vi "Проект квадроКОПТЕР для сравнения.vi"() -> ()   [LabVIEW 2013]
uses:
  <vilib>/Instr/_visa.llb/VISA Configure Serial Port (Instr).vi
  MadgwickOrientationFilter.lvlib
  <vilib>/picture/3D Picture Control/NI_3D Picture Control.lvlib
panel:
  out "Error":u8
  in  "VISA resource name":refnum<visa-resource-name>="COM5"
  out "cluster 2":T1
  out "Error 5":u8 caption="Error"
  in  "Tab Control":enum32{"3D", "Graphs", "U & I", "Out"}(tab)
  out "Scene Display 2":refnum<vi>(3d-picture)
  out "Scene Display":refnum<vi>(3d-picture)
  out "Кватернион":T1(graph)
  out "Q0":sgl
  out "Q1":sgl
  out "Q2":sgl
  out "Q3":sgl
  out "Boolean":bool
  in  "f_cut_diff_vel_xy":dbl
  in  "f_cut_diff_vel_xy b":bool
  in  "f_cut_err_vel_xy":dbl
  in  "f_cut_err_vel_xy b":bool
  in  "KP_Pos_xy b":bool
  in  "KP_Pos_xy":dbl
  in  "KP_Vel_xy b":bool
  in  "KP_Vel_xy":dbl
  in  "KD_Vel_xy":bool
  in  "KD_Vel_xy":dbl
  in  "KI_Acc_xy b":bool
  in  "KI_Vel_xy":dbl
  in  "f_cut_diff_vel_alt":dbl
  in  "f_cut_diff_vel_alt b":bool
  in  "f_cut_err_vel_alt":dbl
  in  "f_cut_diff_acc_alt b":bool
  in  "KI_ugol_z":dbl
  in  "KI_ugol_z_b":bool
  in  "KP_ugol_z":dbl
  in  "KP_ugol_z_b":bool
  in  "KI_rate_z":dbl
  in  "KI_vel_z_b":bool
  in  "KP_rate_z":dbl
  in  "KP_vel_z_b":bool
  in  "KD_rate_z":dbl
  in  "KD_vel_z_b":bool
  in  "KD_vel_xy_b":bool
  in  "KD_rate_xy":dbl
  in  "KI_vel_xy_b":bool
  in  "KP_vel_xy_b":bool
  in  "KI_rate_xy":dbl
  in  "KP_rate_xy":dbl
  in  "KI_ugla_xy_b":bool
  in  "KP_ugla_xy_b":bool
  in  "KI_ugla_xy":dbl
  in  "KP_ugla_xy":dbl
  in  "f_cut_diff":dbl
  in  "f_cut_diff_b":bool
  in  "KP_Pos_alt b":bool
  in  "KP_Pos_alt":dbl
  in  "KP_Vel_alt b":bool
  in  "KP_Vel_alt":dbl
  in  "KD_Vel_alt b":bool
  in  "KD_Vel_alt":dbl
  in  "KP_Acc_alt b":bool
  in  "KP_Acc_alt":dbl
  in  "KI_Acc_alt b":bool
  in  "KI_Vel_alt":dbl
  in  "KD_Acc_alt b":bool
  in  "KD_Acc_alt":dbl
  out "*(type *) &x 11":sgl
  out "*(type *) &x 10":sgl
  out "*(type *) &x 9":sgl
  out "*(type *) &x 8":sgl
  out "sqrt(x)":dbl
  out "unsigned byte array":u8[](array[numeric])
  out "String":string
  out "*(type *) &x 13":sgl
  out "*(type *) &x 12":sgl
  out "*(type *) &x 7":sgl
  out "*(type *) &x 6":sgl
  out "decimated array":u8[](array[numeric])
  out "*(type *) &x 5":sgl
  out "cluster":T1
  in  "stop":bool
  # "346346"
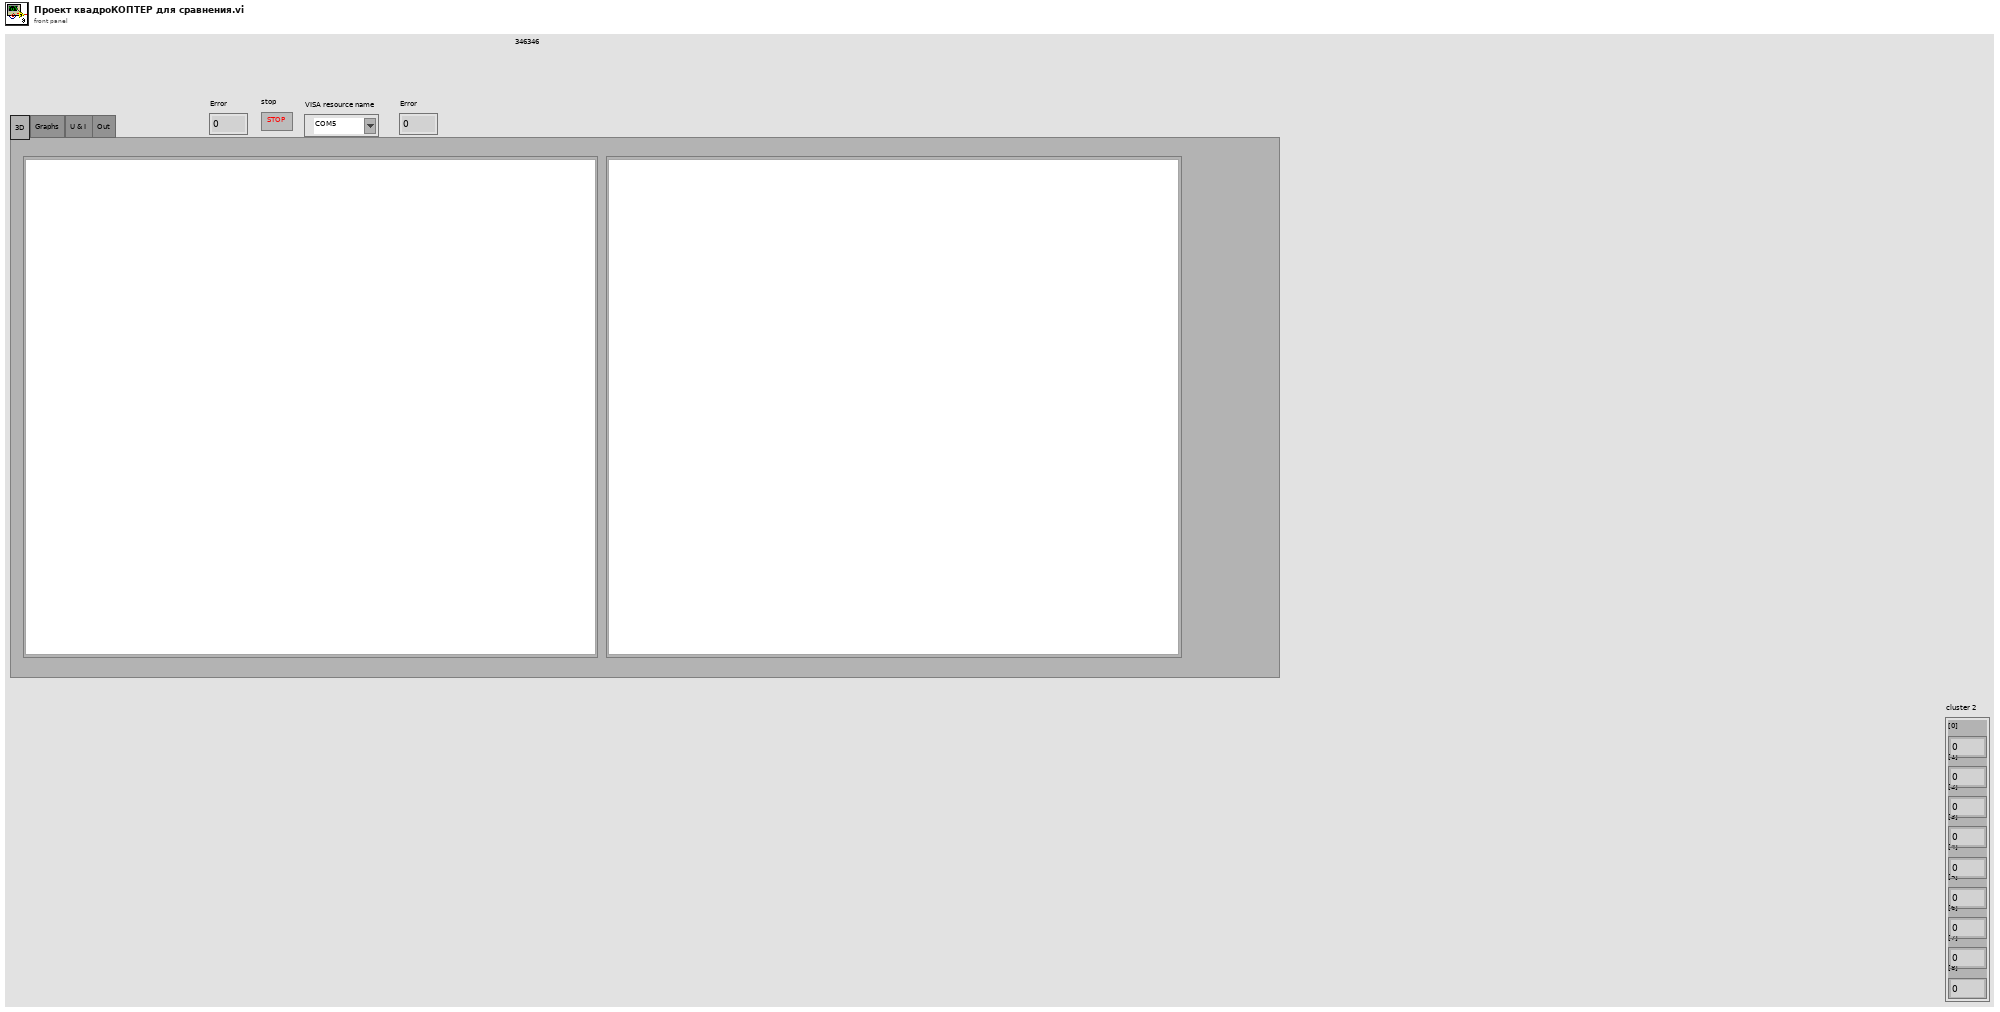
[diagram p1: front panel]
types:
  T1 = cluster{"[0]":dbl, "[1]":dbl, "[2]":dbl, "[3]":dbl, "[4]":dbl, "[5]":dbl, "[6]":dbl, "[7]":dbl, "[8]":dbl}
  T2 = enum16{"open", "replace", "create", "open or create", "replace or create", "replace or create with confirmation"}
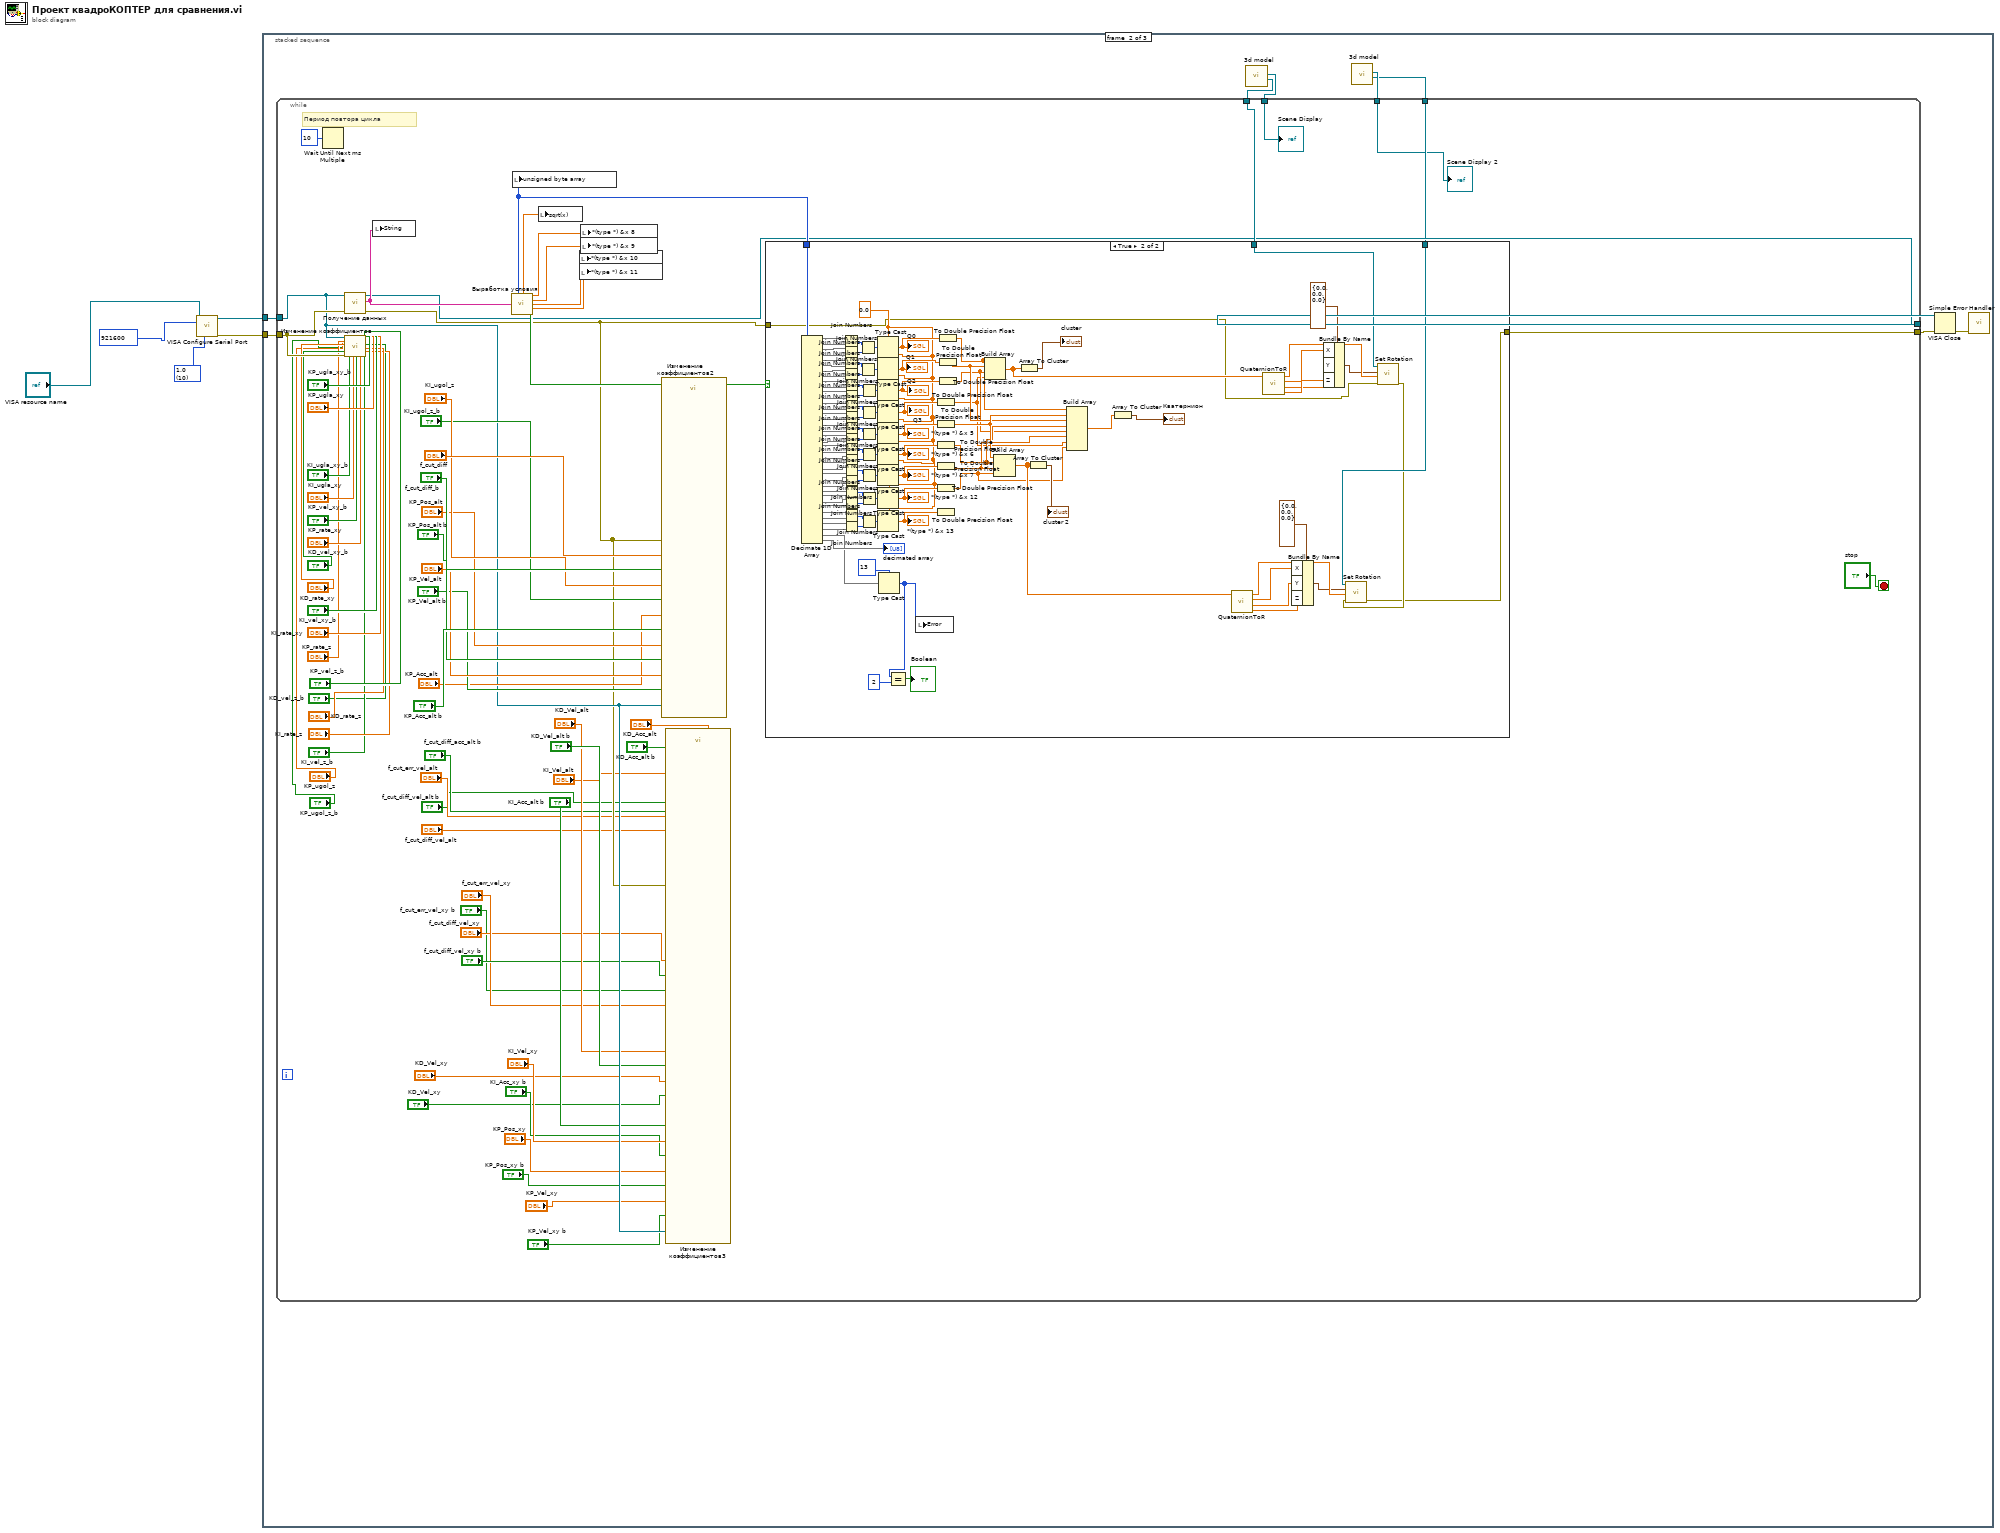
[diagram p0: block diagram]
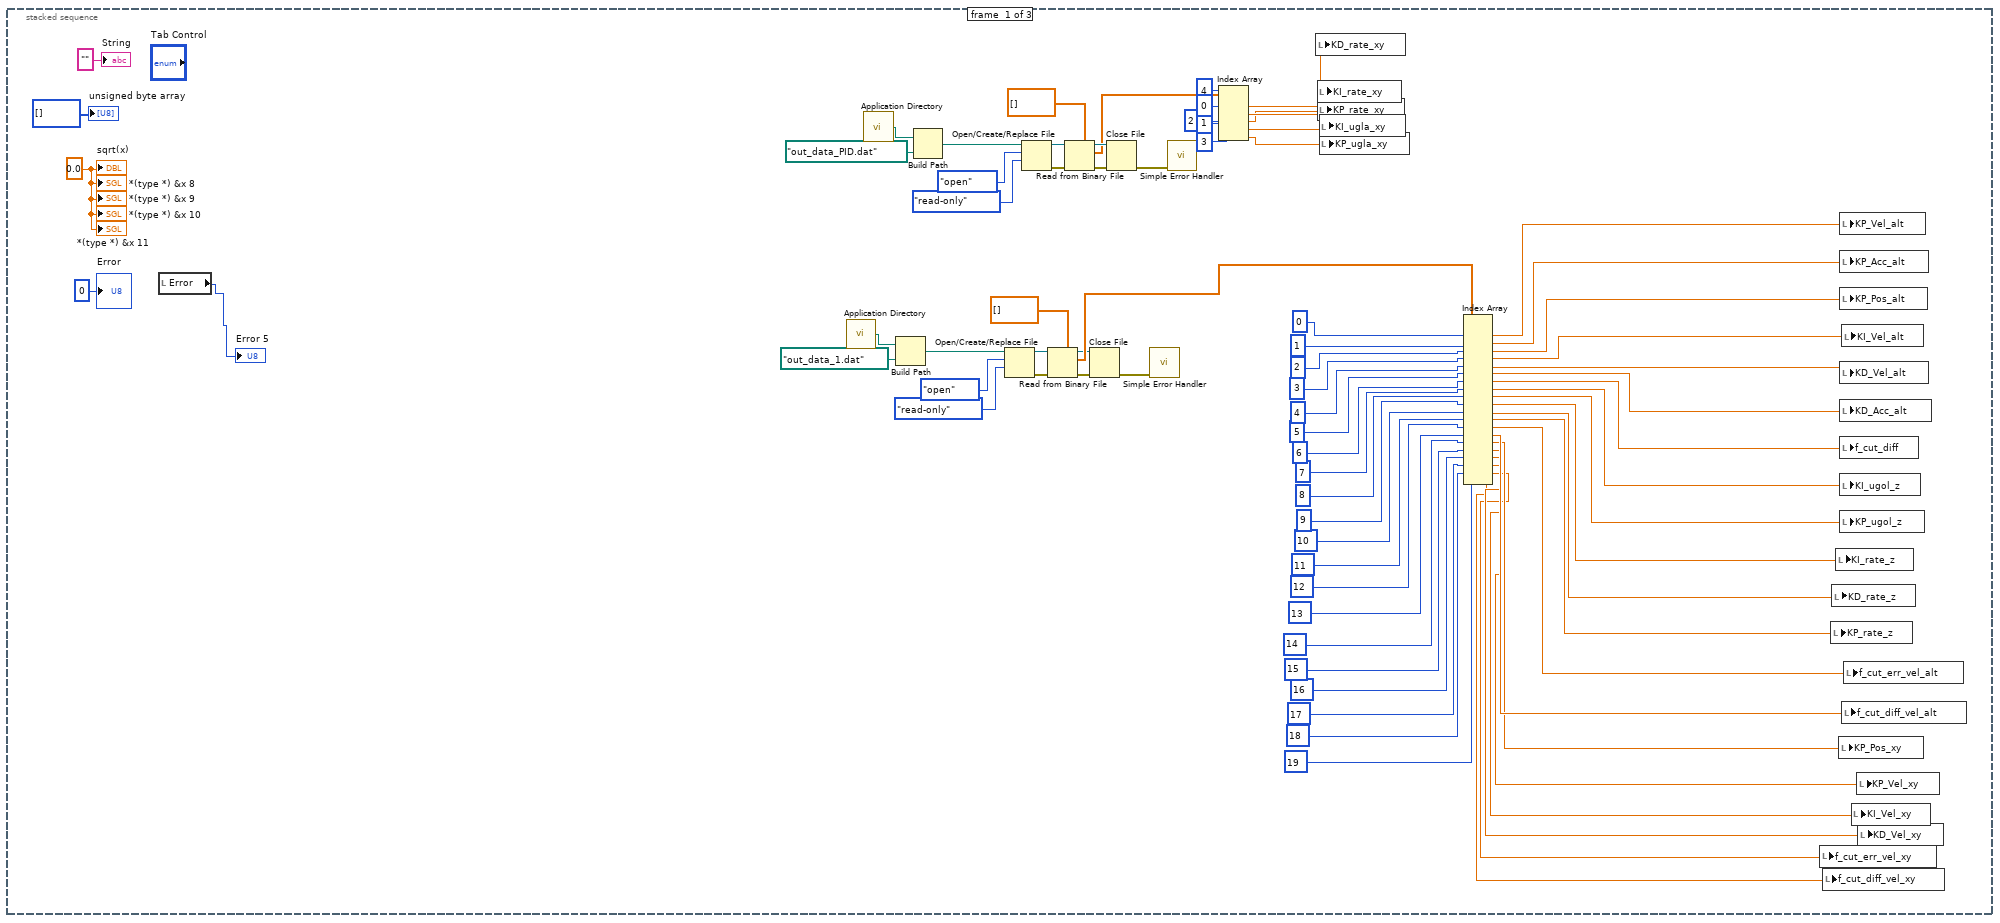
[diagram p2: hidden frame]
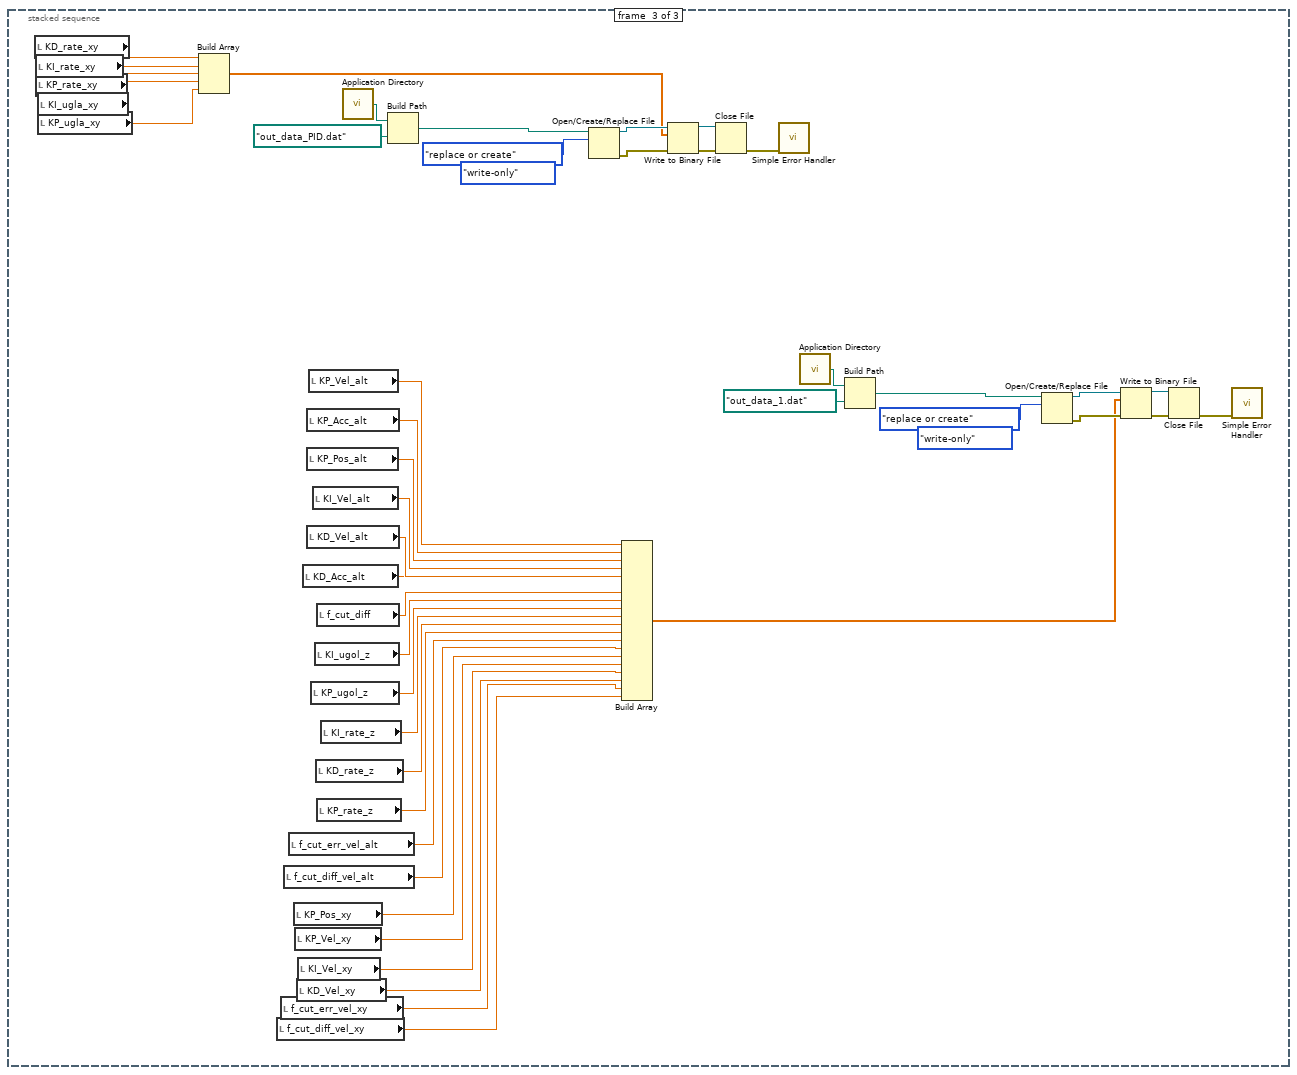
[diagram p4: hidden frame]
diagram:
  w3 = u16 10 items=["1.0"=10, "1.5"=15, "2.0"=20] ("stop bits (10: 1 bit)")
  n1 = call-poly "VISA Configure Serial Port"("VISA resource name"="VISA resource name", "baud rate (9600)"=u32 921600, "stop bits (10: 1 bit)"=w3) -> ("VISA resource name out"=w5:refnum<visa-resource-name>, "error out"=w4:errorcluster)  [unwired: 11 in]
  n2 = stacked-sequence {
    tunnel: w5 -> [_ w93 _]
    tunnel: w4 -> [_ w91 _]
    frame #0 {
      w82 = 0.0 ("sqrt(x)")
      n3 = local read "Error"() -> (→"Error 5":u8)
      n4 = call <vilib>:"Application Directory.vi"() -> ("Application Directory"=w56:path)
      n5 = call <vilib>:"Application Directory.vi"() -> ("Application Directory"=w74:path)
      n6 = Build Path(base path=w56, name or relative path=path "out_data_1.dat" ("default name")) -> (appended path=w52:path)
      n7 = Build Path(base path=w74, name or relative path=path "out_data_PID.dat" ("default name")) -> (appended path=w78:path)
      n8 = Open/Create/Replace File(file path (use dialog)=w52, operation (0:open)=T2."open", access (0:read/write)=enum16{"read/write", "read-only", "write-only"}."read-only") -> (refnum out=w57:refnum<file>, error out=w58:errorcluster)  [unwired: 3 in, 1 out]
      n9 = Open/Create/Replace File(file path (use dialog)=w78, operation (0:open)=T2."open", access (0:read/write)=enum16{"read/write", "read-only", "write-only"}."read-only") -> (refnum out=w73:refnum<file>, error out=w72:errorcluster)  [unwired: 3 in, 1 out]
      n10 = Read from Binary File(5:dbl[] [] ("appended array"), 8:w58, 11:w57) -> (0:w60:errorcluster, 2:w62:dbl[], 3:w59:refnum<file>)  [unwired: 3 in, 1 out]
      n11 = Read from Binary File(5:dbl[] [] ("appended array"), 8:w72, 11:w73) -> (0:w70:errorcluster, 2:w68:dbl[], 3:w71:refnum<file>)  [unwired: 3 in, 1 out]
      n12 = Close File(refnum=w59, error in=w60) -> (error out=w51:errorcluster)  [unwired: 1 out]
      n13 = Close File(refnum=w71, error in=w70) -> (error out=w79:errorcluster)  [unwired: 1 out]
      n14 = call <vilib>:"Simple Error Handler.vi"("error in (no error)"=w51) -> ()  [unwired: 4 in, 5 out]
      n15 = call <vilib>:"Simple Error Handler.vi"("error in (no error)"=w79) -> ()  [unwired: 4 in, 5 out]
      n16 = Index Array(array=w68, index #1=0 ("index"), index #2=1 ("index"), index #3=2 ("index"), index #4=3 ("index"), index #5=4 ("index")) -> (element #1=w50:dbl, element #2=w49:dbl, element #3=w48:dbl, element #4=w47:dbl, element #5=w46:dbl)
      n17 = local write "KD_rate_xy"(w50) -> ()
      n18 = local write "KI_rate_xy"(w49) -> ()
      n19 = local write "KP_rate_xy"(w48) -> ()
      n20 = local write "KI_ugla_xy"(w47) -> ()
      n21 = local write "KP_ugla_xy"(w46) -> ()
      n22 = Index Array(array=w62, index #1=0 ("index"), index #2=1 ("index"), index #3=2 ("index"), index #4=3 ("index"), index #5=4 ("index"), index #6=5 ("index"), index #7=6 ("index"), index #8=7 ("index"), index #9=8 ("index"), index #10=9 ("index"), index #11=10 ("index"), index #12=11 ("index"), index #13=12 ("index"), index #14=13 ("index"), index #15=14 ("index"), index #16=15 ("index"), index #17=16 ("index"), index #18=17 ("index"), index #19=18 ("index"), index #20=19 ("index")) -> (element #1=w45:dbl, element #2=w44:dbl, element #3=w43:dbl, element #4=w42:dbl, element #5=w41:dbl, element #6=w40:dbl, element #7=w39:dbl, element #8=w38:dbl, element #9=w37:dbl, element #10=w36:dbl, element #11=w35:dbl, element #12=w34:dbl, element #13=w19:dbl, element #14=w18:dbl, element #15=w11:dbl, element #16=w10:dbl, element #17=w9:dbl, element #18=w8:dbl, element #19=w7:dbl, element #20=w6:dbl)
      n23 = local write "f_cut_err_vel_xy"(w7) -> ()
      n24 = local write "f_cut_diff_vel_xy"(w6) -> ()
      n25 = local write "KP_rate_z"(w34) -> ()
      n26 = local write "KD_rate_z"(w35) -> ()
      n27 = local write "KI_rate_z"(w36) -> ()
      n28 = local write "KP_Pos_xy"(w11) -> ()
      n29 = local write "KP_Vel_alt"(w45) -> ()
      n30 = local write "KP_Acc_alt"(w44) -> ()
      n31 = local write "KP_Pos_alt"(w43) -> ()
      n32 = local write "KD_Vel_alt"(w41) -> ()
      n33 = local write "KD_Acc_alt"(w40) -> ()
      n34 = local write "f_cut_diff"(w39) -> ()
      n35 = local write "KI_ugol_z"(w38) -> ()
      n36 = local write "KP_ugol_z"(w37) -> ()
      n37 = local write "KI_Vel_alt"(w42) -> ()
      n38 = local write "f_cut_diff_vel_alt"(w18) -> ()
      n39 = local write "f_cut_err_vel_alt"(w19) -> ()
      n40 = local write "KI_Vel_xy"(w9) -> ()
      n41 = local write "KP_Vel_xy"(w10) -> ()
      n42 = local write "KD_Vel_xy"(w8) -> ()
      "String" <- "" ("String")
      "unsigned byte array" <- u8[] [] ("unsigned byte array")
      "sqrt(x)" <- w82
      "*(type *) &x 8" <- w82
      "*(type *) &x 9" <- w82
      "*(type *) &x 10" <- w82
      "*(type *) &x 11" <- w82
      "Error" <- u8 0 ("Error")
    }
    frame #1 {
      n43 = call "3d model.vi"() -> ("Коптер + оси"=w88:refnum<vi>, "Вся сцена"=w89:refnum<vi>)  [unwired: 9 in, 1 out]
      n44 = call "3d model.vi"() -> ("Коптер + оси"=w85:refnum<vi>, "Вся сцена"=w86:refnum<vi>)  [unwired: 9 in, 1 out]
      n45 = while {
        tunnel: w93 -> [w119]
        tunnel: [w130] -> w92
        tunnel: w91 -> [w159]
        tunnel: [w149] -> w90
        tunnel: w89 -> [w160]
        tunnel: w88 -> [w158]
        tunnel: w86 -> [w94]
        tunnel: w85 -> [w95]
        stop <- "stop" stop-if-true
        # "Период повтора цикла"
        n46 = Wait Until Next ms Multiple(millisecond multiple=u32 10) -> ()  [unwired: 1 out]
        n47 = call "Получение данных.vi"("error in (no error)"=w159, "VISA Refnum in"=w119) -> ("error out"=w118:errorcluster, "String"=w156:string, "VISA Refnum out"=w130:refnum<visa-resource-name>)  [unwired: 7 in]
        n48 = call "Изменение коэффициентов.vi"("VISA Refnum in"=w119, "KP_ugol_z"="KP_ugol_z", "KD_vel"="KD_rate_xy", "KP_ugol_z_b"="KP_ugol_z_b", "KD_vel 2"="KD_vel_xy_b", "error in (no error)"=w159, "KI_vel 2"="KI_vel_xy_b", "KI_ugla 2"="KI_ugla_xy_b", "KP_ugla"="KP_ugla_xy", "KI_ugla"="KI_ugla_xy", "KP_ugla 2"="KP_ugla_xy_b", "KP_vel 2"="KP_vel_xy_b", "KI_vel"="KI_rate_xy", "KP_vel"="KP_rate_xy", "KP_vel_z_b"="KP_vel_z_b", "KP_vel_z"="KP_rate_z", "KD_vel_z_b"="KD_vel_z_b", "KD_vel_z"="KD_rate_z", "KI_vel_z"="KI_rate_z", "KI_vel_z_b"="KI_vel_z_b") -> ()
        n49 = local write "String"(w156) -> ()
        n50 = call "Выработка условия.vi"("String"=w156) -> ("unsigned byte array"=w155:u8[], "sqrt(x)"=w154:dbl, "*(type *) &x 8"=w153:sgl, "*(type *) &x 9"=w152:sgl, "*(type *) &x 10"=w151:sgl, "*(type *) &x 11"=w150:sgl, "Boolean"=w157:bool)  [unwired: 8 in]
        n51 = local write "unsigned byte array"(w155) -> ()
        n52 = local write "sqrt(x)"(w154) -> ()
        n53 = local write "*(type *) &x 10"(w151) -> ()
        n54 = local write "*(type *) &x 11"(w150) -> ()
        n55 = local write "*(type *) &x 8"(w153) -> ()
        n56 = local write "*(type *) &x 9"(w152) -> ()
        n57 = call "Изменение коэффициентов2.vi"("KI_ugol_z_b"="KI_ugol_z_b", "KI_ugol_z"="KI_ugol_z", "f_cut_diff_b"="f_cut_diff_b", "f_cut_diff"="f_cut_diff", "KP_Pos_alt b"="KP_Pos_alt b", "KP_Pos_alt"="KP_Pos_alt", "KP_Vel_alt b"="KP_Vel_alt b", "KP_Vel_alt"="KP_Vel_alt", "VISA Refnum in"=w119, "error in (no error)"=w118, "KP_Acc_alt b"="KP_Acc_alt b", "KP_Acc_alt"="KP_Acc_alt") -> ()  [unwired: 16 in]
        n58 = call "Изменение коэффициентов3.vi"("VISA Refnum in"=w119, "error in (no error)"=w118, "f_cut_diff_vel_xy b"="f_cut_diff_vel_xy b", "KP_Pos_xy b"="KP_Pos_xy b", "KD_Vel_alt b"="KD_Vel_alt b", "KD_Vel_alt"="KD_Vel_alt", "f_cut_err_vel_xy"="f_cut_err_vel_xy", "KI_Acc_alt b"="KI_Acc_alt b", 8:"KD_Vel_xy"="KD_Vel_xy", "KP_Pos_xy"="KP_Pos_xy", "f_cut_err_vel_xy b"="f_cut_err_vel_xy b", "f_cut_diff_vel_xy"="f_cut_diff_vel_xy", 12:"KD_Vel_xy"="KD_Vel_xy", "KP_Vel_xy b"="KP_Vel_xy b", "KI_Vel_xy"="KI_Vel_xy", "f_cut_diff_vel_alt"="f_cut_diff_vel_alt", "KI_Vel_xy b"="KI_Acc_xy b", "f_cut_diff_vel_alt b"="f_cut_diff_vel_alt b", "KI_Acc_alt"="KI_Vel_alt", "KD_Acc_alt b"="KD_Acc_alt b", "KP_Vel_xy"="KP_Vel_xy", "KD_Acc_alt"="KD_Acc_alt", "f_cut_diff_acc_alt b"="f_cut_diff_acc_alt b", "f_cut_diff_acc_alt"="f_cut_err_vel_alt") -> ()  [unwired: 4 in]
        n59 = case shown="True" w157 {
          tunnel: w155 -> [_ w232]
          tunnel: w158 -> [_ w188]
          tunnel: w118 -> [w163 w186]
          tunnel: [w163 w176] -> w149
          tunnel: w95 -> [_ w179]
          frame False {
          }
          frame True {
            w193 = sgl 0.0
            n60 = Decimate 1D Array(w232) -> (w239:u8[], w240:u8[], w241:u8[], w242:u8[], w247:u8[], w248:u8[], w249:u8[], w250:u8[], w255:u8[], w256:u8[], w257:u8[], w258:u8[], w259:u8[], w260:u8[], w261:u8[], w262:u8[], w270:u8[], w271:u8[], w272:u8[], w273:u8[], w223:u8[], w222:u8[], w221:u8[], w220:u8[], w219:u8[], w218:u8[], w217:u8[], w216:u8[], w206:u8[], w205:u8[], w204:u8[], w203:u8[], w197:u8[], w196:u8[], w195:u8[], w194:u8[], w192:u8[], →"decimated array":u8[])
            n61 = Join Numbers(hi=w239, lo=w240) -> ((hi.lo)=w243:u16[])
            n62 = Join Numbers(hi=w241, lo=w242) -> ((hi.lo)=w244:u16[])
            n63 = Join Numbers(hi=w247, lo=w248) -> ((hi.lo)=w245:u16[])
            n64 = Join Numbers(hi=w249, lo=w250) -> ((hi.lo)=w246:u16[])
            n65 = Join Numbers(hi=w255, lo=w256) -> ((hi.lo)=w251:u16[])
            n66 = Join Numbers(hi=w257, lo=w258) -> ((hi.lo)=w252:u16[])
            n67 = Join Numbers(hi=w259, lo=w260) -> ((hi.lo)=w253:u16[])
            n68 = Join Numbers(hi=w261, lo=w262) -> ((hi.lo)=w254:u16[])
            n69 = Join Numbers(hi=w270, lo=w271) -> ((hi.lo)=w267:u16[])
            n70 = Join Numbers(hi=w272, lo=w273) -> ((hi.lo)=w268:u16[])
            n71 = Join Numbers(hi=w223, lo=w222) -> ((hi.lo)=w228:u16[])
            n72 = Join Numbers(hi=w221, lo=w220) -> ((hi.lo)=w229:u16[])
            n73 = Join Numbers(hi=w219, lo=w218) -> ((hi.lo)=w224:u16[])
            n74 = Join Numbers(hi=w217, lo=w216) -> ((hi.lo)=w225:u16[])
            n75 = Join Numbers(hi=w206, lo=w205) -> ((hi.lo)=w207:u16[])
            n76 = Join Numbers(hi=w204, lo=w203) -> ((hi.lo)=w208:u16[])
            n77 = Join Numbers(hi=w197, lo=w196) -> ((hi.lo)=w198:u16[])
            n78 = Join Numbers(hi=w195, lo=w194) -> ((hi.lo)=w199:u16[])
            n79 = Join Numbers(hi=w243, lo=w244) -> ((hi.lo)=w263:u32[])
            n80 = Join Numbers(hi=w245, lo=w246) -> ((hi.lo)=w215:u32[])
            n81 = Join Numbers(hi=w251, lo=w252) -> ((hi.lo)=w264:u32[])
            n82 = Join Numbers(hi=w253, lo=w254) -> ((hi.lo)=w265:u32[])
            n83 = Join Numbers(hi=w267, lo=w268) -> ((hi.lo)=w269:u32[])
            n84 = Join Numbers(hi=w228, lo=w229) -> ((hi.lo)=w230:u32[])
            n85 = Join Numbers(hi=w224, lo=w225) -> ((hi.lo)=w226:u32[])
            n86 = Join Numbers(hi=w207, lo=w208) -> ((hi.lo)=w209:u32[])
            n87 = Join Numbers(hi=w198, lo=w199) -> ((hi.lo)=w200:u32[])
            n88 = Type Cast(type=w193, x=w263) -> (*(type *) &x=w211:sgl)
            "Q0" <- w211
            n89 = Type Cast(type=w193, x=w215) -> (*(type *) &x=w212:sgl)
            "Q1" <- w212
            n90 = Type Cast(type=w193, x=w264) -> (*(type *) &x=w213:sgl)
            "Q2" <- w213
            n91 = Type Cast(type=w193, x=w265) -> (*(type *) &x=w214:sgl)
            "Q3" <- w214
            n92 = Type Cast(type=w193, x=w269) -> (*(type *) &x=w274:sgl)
            "*(type *) &x 5" <- w274
            n93 = Type Cast(type=w193, x=w230) -> (*(type *) &x=w231:sgl)
            "*(type *) &x 6" <- w231
            n94 = Type Cast(type=w193, x=w226) -> (*(type *) &x=w227:sgl)
            "*(type *) &x 7" <- w227
            n95 = Type Cast(type=w193, x=w209) -> (*(type *) &x=w202:sgl)
            "*(type *) &x 12" <- w202
            n96 = Type Cast(type=w193, x=w200) -> (*(type *) &x=w201:sgl)
            "*(type *) &x 13" <- w201
            n97 = Type Cast(type=u8 13 ("y"), x=w192) -> (*(type *) &x=w187:u8)
            n98 = Equal?(x=w187, y=u8 2) -> (x = y?=→"Boolean":bool)
            n99 = local write "Error"(w187) -> ()
            n100 = To Double Precision Float(number=w214) -> (double precision float=w165:dbl)
            n101 = To Double Precision Float(number=w274) -> (double precision float=w170:dbl)
            n102 = To Double Precision Float(number=w231) -> (double precision float=w168:dbl)
            n103 = To Double Precision Float(number=w227) -> (double precision float=w166:dbl)
            n104 = To Double Precision Float(number=w202) -> (double precision float=w164:dbl)
            n105 = To Double Precision Float(number=w201) -> ()  [unwired: 1 out]
            n106 = To Double Precision Float(number=w211) -> (double precision float=w171:dbl)
            n107 = To Double Precision Float(number=w212) -> (double precision float=w169:dbl)
            n108 = To Double Precision Float(number=w213) -> (double precision float=w167:dbl)
            n109 = Build Array(w171, w169, w167, w165) -> (w266:dbl[])
            n110 = Build Array(w170, w168, w166, w164) -> (w180:dbl[])
            n111 = Array To Cluster(array=w266) -> (cluster=→"cluster":T1)
            n112 = Array To Cluster(array=w180) -> (cluster=→"cluster 2":T1)
            n113 = Build Array(w171, w170, w169, w168, w167, w166, w165, w164) -> (w174:dbl[])
            n114 = Array To Cluster(array=w174) -> (cluster=→"Кватернион":T1)
            n115 = call "QuaternionToR.vi"("Quaternion"=w180) -> ("Rz"=w178:dbl, "Ry"=w182:dbl, "Rx"=w181:dbl, "Theta"=w185:dbl)  [unwired: 7 in]
            n116 = call "QuaternionToR.vi"("Quaternion"=w266) -> ("Rz"=w235:dbl, "Ry"=w234:dbl, "Rx"=w233:dbl, "Theta"=w238:dbl)  [unwired: 7 in]
            n117 = Bundle By Name(cluster=cluster{"X":sgl, "Y":sgl, "Z":sgl} {"X"=0.0, "Y"=0.0, "Z"=0.0} ("Axis"), "X"=w181, "Y"=w182, "Z"=w178) -> (w183:cluster{"X":sgl, "Y":sgl, "Z":sgl})
            n118 = Bundle By Name(cluster=cluster{"X":sgl, "Y":sgl, "Z":sgl} {"X"=0.0, "Y"=0.0, "Z"=0.0} ("Axis"), "X"=w233, "Y"=w234, "Z"=w235) -> (w236:cluster{"X":sgl, "Y":sgl, "Z":sgl})
            n119 = call <vilib>:"Set Rotation.vi"("error in (no error)"=w186, "Angle"=w238, "Axis"=w236, "Scene Object"=w188) -> ("error out"=w177:errorcluster)  [unwired: 6 in, 1 out]
            n120 = call <vilib>:"Set Rotation.vi"("error in (no error)"=w177, "Angle"=w185, "Axis"=w183, "Scene Object"=w179) -> ("error out"=w176:errorcluster)  [unwired: 6 in, 1 out]
          }
        }
        "Scene Display" <- w160
        "Scene Display 2" <- w94
      }
      n121 = VISA Close(VISA resource name=w92, error in (no error)=w90) -> (error out=w87:errorcluster)
      n122 = call <vilib>:"Simple Error Handler.vi"("error in (no error)"=w87) -> ()  [unwired: 4 in, 5 out]
    }
    frame #2 {
      (unwired) enum16{"read/write", "read-only", "write-only"}."write-only" ("access (0:read/write)")
      (unwired) enum16{"read/write", "read-only", "write-only"}."write-only" ("access (0:read/write)")
      n123 = local read "KD_rate_xy"() -> (w319:dbl)
      n124 = local read "KI_rate_xy"() -> (w318:dbl)
      n125 = local read "KP_rate_xy"() -> (w317:dbl)
      n126 = local read "KI_ugla_xy"() -> (w316:dbl)
      n127 = local read "KP_ugla_xy"() -> (w315:dbl)
      n128 = Build Array(w319, w318, w317, w316, w315) -> (w305:dbl[])
      n129 = local read "f_cut_diff_vel_xy"() -> (w275:dbl)
      n130 = local read "f_cut_err_vel_xy"() -> (w276:dbl)
      n131 = local read "f_cut_diff_vel_alt"() -> (w281:dbl)
      n132 = local read "f_cut_err_vel_alt"() -> (w282:dbl)
      n133 = local read "KP_Pos_xy"() -> (w280:dbl)
      n134 = local read "KP_Vel_xy"() -> (w279:dbl)
      n135 = local read "KD_Vel_xy"() -> (w277:dbl)
      n136 = local read "KI_Vel_xy"() -> (w278:dbl)
      n137 = local read "KD_Acc_alt"() -> (w290:dbl)
      n138 = local read "KP_Acc_alt"() -> (w294:dbl)
      n139 = local read "KP_Pos_alt"() -> (w293:dbl)
      n140 = local read "KD_Vel_alt"() -> (w291:dbl)
      n141 = local read "KP_Vel_alt"() -> (w295:dbl)
      n142 = local read "KP_ugol_z"() -> (w287:dbl)
      n143 = local read "KI_Vel_alt"() -> (w292:dbl)
      n144 = local read "KI_ugol_z"() -> (w288:dbl)
      n145 = local read "KD_rate_z"() -> (w285:dbl)
      n146 = local read "f_cut_diff"() -> (w289:dbl)
      n147 = local read "KP_rate_z"() -> (w284:dbl)
      n148 = local read "KI_rate_z"() -> (w286:dbl)
      n149 = call <vilib>:"Application Directory.vi"() -> ("Application Directory"=w312:path)
      n150 = Build Path(base path=w312, name or relative path=path "out_data_PID.dat" ("default name")) -> (appended path=w314:path)
      n151 = Open/Create/Replace File(file path (use dialog)=w314, operation (0:open)=T2."replace or create") -> (refnum out=w307:refnum<file>, error out=w306:errorcluster)  [unwired: 4 in, 1 out]
      n152 = Build Array(w295, w294, w293, w292, w291, w290, w289, w288, w287, w286, w285, w284, w282, w281, w280, w279, w278, w277, w276, w275) -> (w283:dbl[])
      n153 = Write to Binary File(file (use dialog)=w307, data=w305, error in=w306) -> (refnum out=w308:refnum<file>, error out=w309:errorcluster)  [unwired: 3 in, 1 out]
      n154 = Close File(refnum=w308, error in=w309) -> (error out=w310:errorcluster)  [unwired: 1 out]
      n155 = call <vilib>:"Simple Error Handler.vi"("error in (no error)"=w310) -> ()  [unwired: 4 in, 5 out]
      n156 = call <vilib>:"Application Directory.vi"() -> ("Application Directory"=w298:path)
      n157 = Build Path(base path=w298, name or relative path=path "out_data_1.dat" ("default name")) -> (appended path=w296:path)
      n158 = Open/Create/Replace File(file path (use dialog)=w296, operation (0:open)=T2."replace or create") -> (refnum out=w303:refnum<file>, error out=w304:errorcluster)  [unwired: 4 in, 1 out]
      n159 = Write to Binary File(file (use dialog)=w303, data=w283, error in=w304) -> (refnum out=w302:refnum<file>, error out=w301:errorcluster)  [unwired: 3 in, 1 out]
      n160 = Close File(refnum=w302, error in=w301) -> (error out=w300:errorcluster)  [unwired: 1 out]
      n161 = call <vilib>:"Simple Error Handler.vi"("error in (no error)"=w300) -> ()  [unwired: 4 in, 5 out]
    }
  }
